vi "Read Scale.vi"(8 "error in (no error)":errorcluster, 11 "AI in":refnum<class "AI.lvclass">) -> (0 "error out":errorcluster, 2 "Scale_PiecedLinear.lvclass":refnum<class "Scale_PiecedLinear.lvclass">, 3 "AI out":refnum<class "AI.lvclass">)   [LabVIEW 2019, in "AI.lvclass"]
uses:
  AI.lvclass
  PiecedLinearScale_class/Scale_PiecedLinear.lvclass
  AI.lvclass/AI.ctl
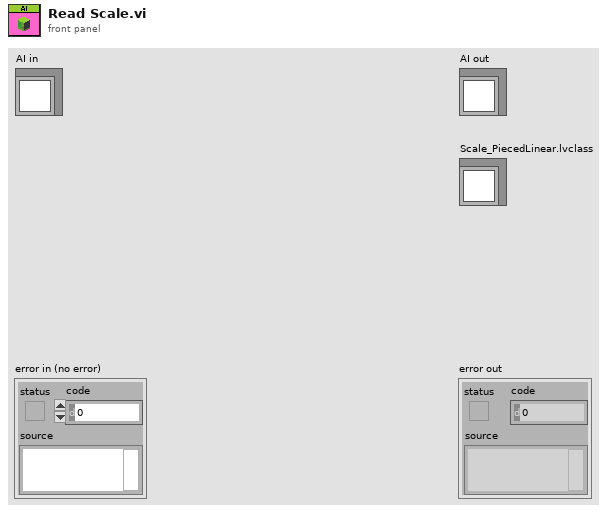
[diagram p1: front panel]
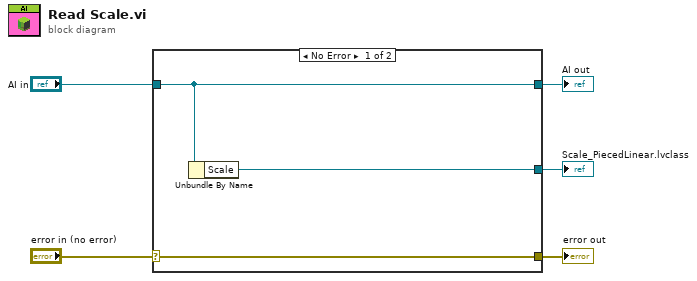
[diagram p0: block diagram]
diagram:
  n1 = case shown="No Error" "error in (no error)" {
    selector: "error in (no error)" -> [w8 w9]
    tunnel: [w8 w9] -> w4
    tunnel: [w7 w10] -> w2
    tunnel: "AI in" -> [w7 w10]
    tunnel: [w6 _] -> w1
    frame No Error {
      n2 = Unbundle By Name(w7) -> ("Scale"=w6:refnum<class "Scale_PiecedLinear.lvclass">)
    }
    frame Error {
    }
  }
  "error out" <- w4
  "AI out" <- w2
  "Scale_PiecedLinear.lvclass" <- w1
